vi "Message Handler (reentrant).vi"(7 "MsgQ Name":string, 8 "error in (no error)":errorcluster, 10 "Message to send":T1, 11 "Mode":T2) -> (0 "error out":errorcluster, 1 "Message Recieved?":bool, 2 "Message recieved":T1, 3 "Queue Names":string[](array[string]))   [LabVIEW 2013, in "Interloop MessageQ.lvlib"]
doc: "Keeps track of all message queues. Modes of operation : initialize, close, create queue, destroy queue, send message, Broadcase message (sends to queues excluding the passed in queue) read message. This vi should not block and controls access to messaging.\nReentrant must be wrapped for each message queue used in an application. Wrapper allows for create, send to read from, kill and broadcast."
uses:
  Interloop MessageQ.lvlib
  Message queue handler mode enums.ctl
  Message cluster.ctl
  Message Queue Ref.ctl
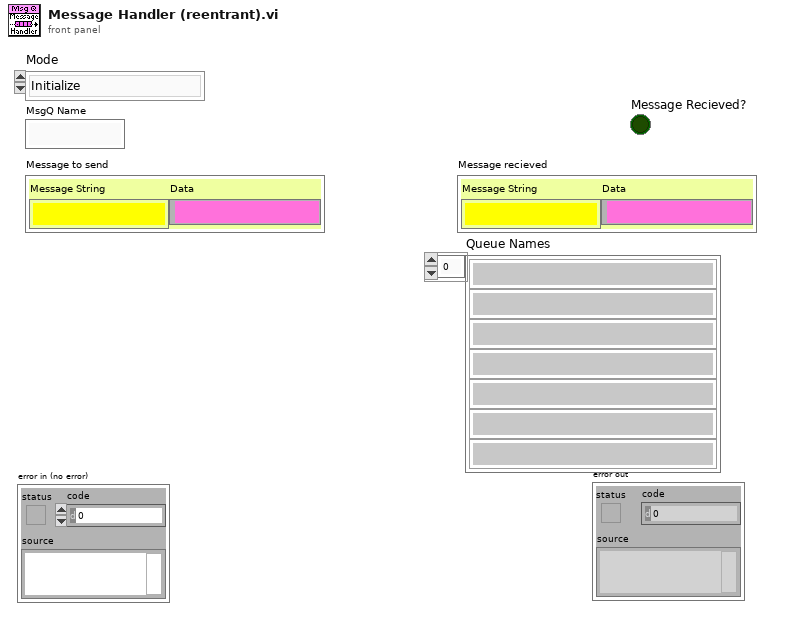
[diagram p1: front panel]
types:
  T1 = typedef "Interloop MessageQ.lvlib/Message cluster.ctl" = cluster{"Message String":string, "Data":variant}
  T2 = typedef "Interloop MessageQ.lvlib/Message queue handler mode enums.ctl" = enum16{"Initialize", "Create MsgQ", "Destroy MsgQ", "Send Message", "Broadcast Message", "Read Message", "Close"}
  T3 = typedef "Interloop MessageQ.lvlib/Message Queue Ref.ctl" = refnum<queue>
  T4 = typedef "Message cluster.ctl" = cluster{"Message String":string, "Data":variant}
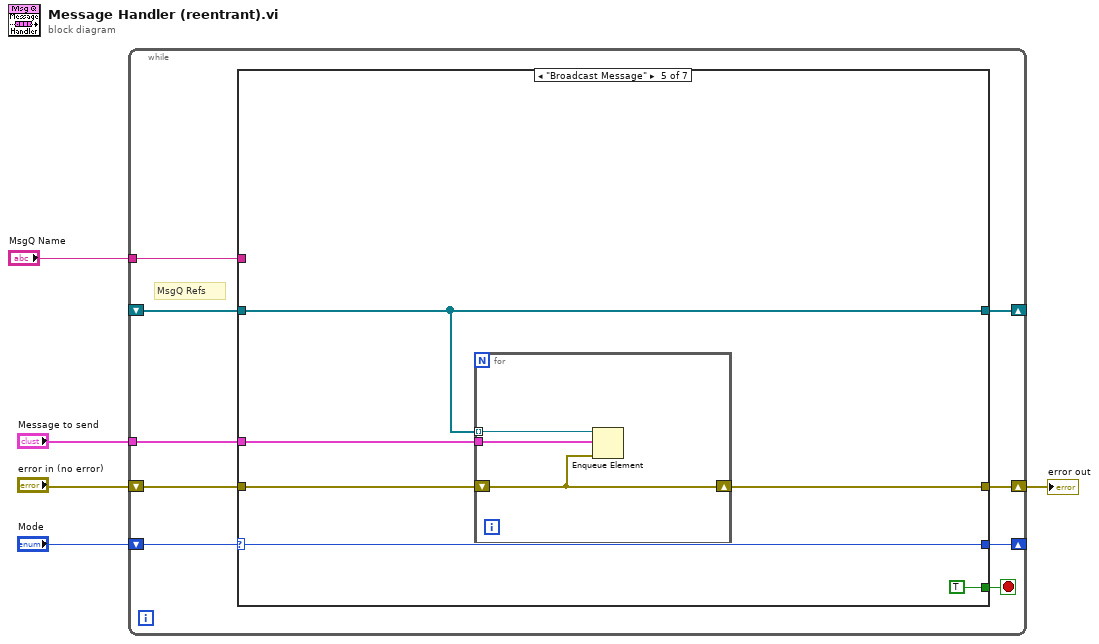
[diagram p0: block diagram]
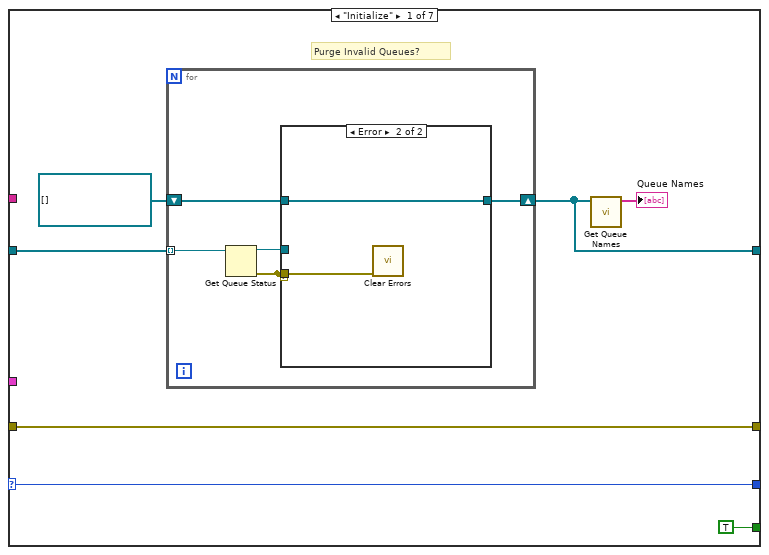
[diagram p2: hidden frame]
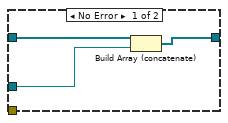
[diagram p3: hidden frame]
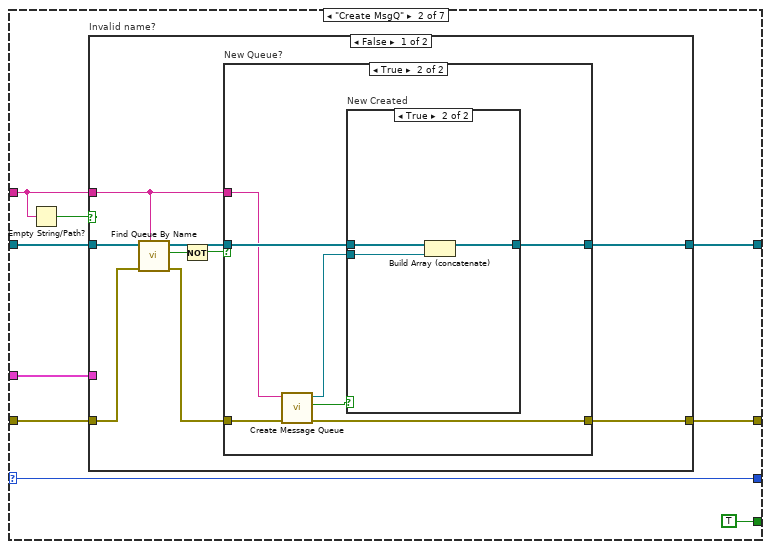
[diagram p4: hidden frame]
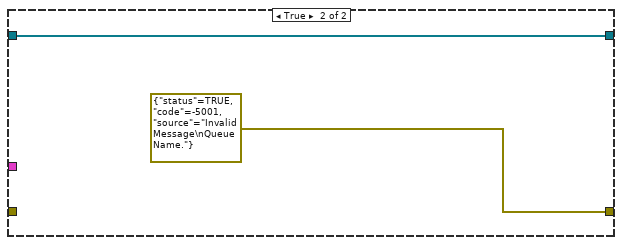
[diagram p7: hidden frame]
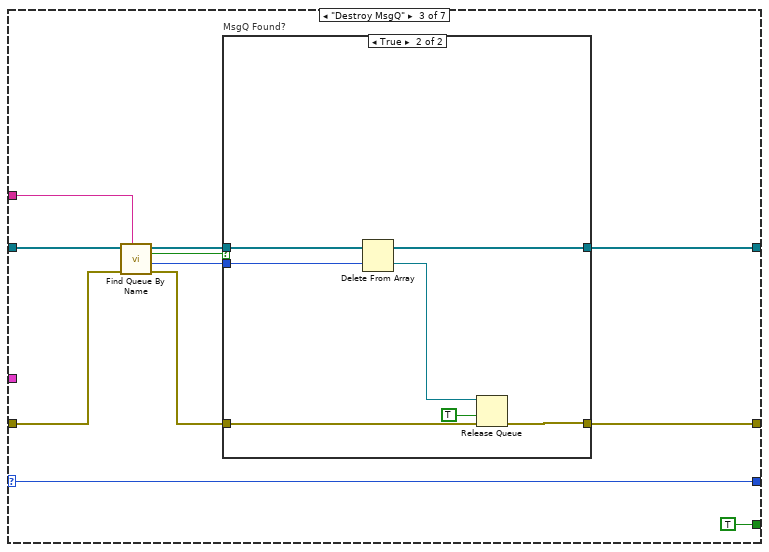
[diagram p8: hidden frame]
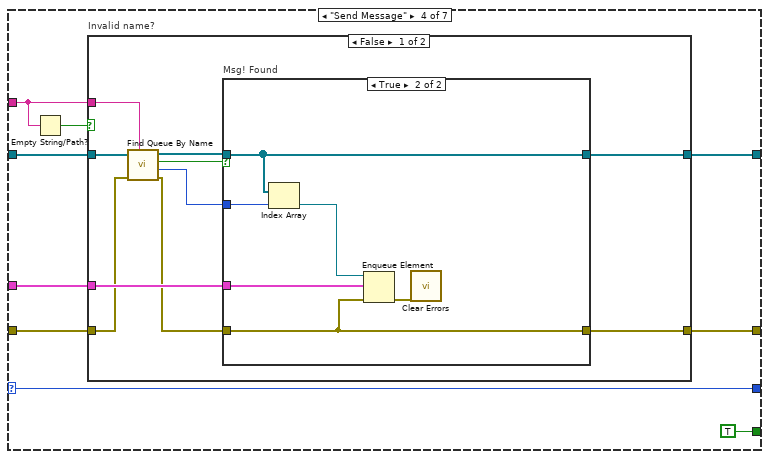
[diagram p10: hidden frame]
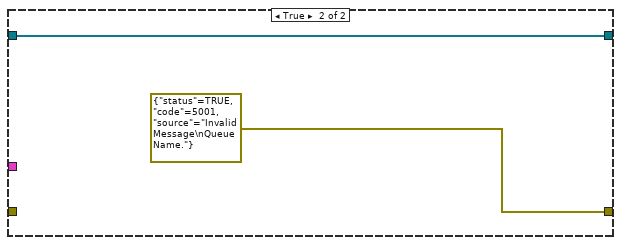
[diagram p12: hidden frame]
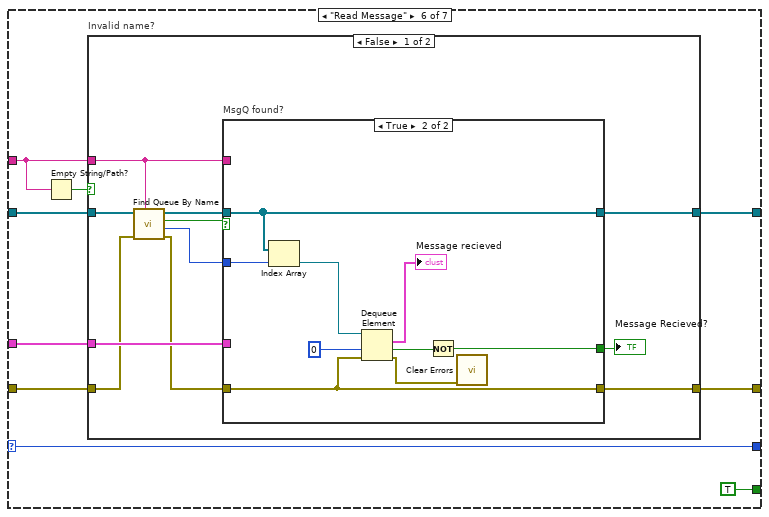
[diagram p13: hidden frame]
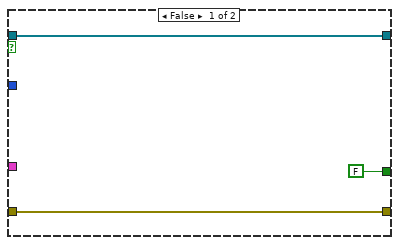
[diagram p14: hidden frame]
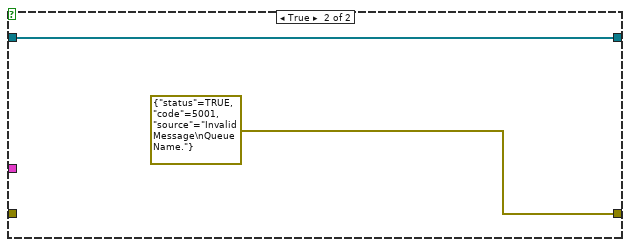
[diagram p15: hidden frame]
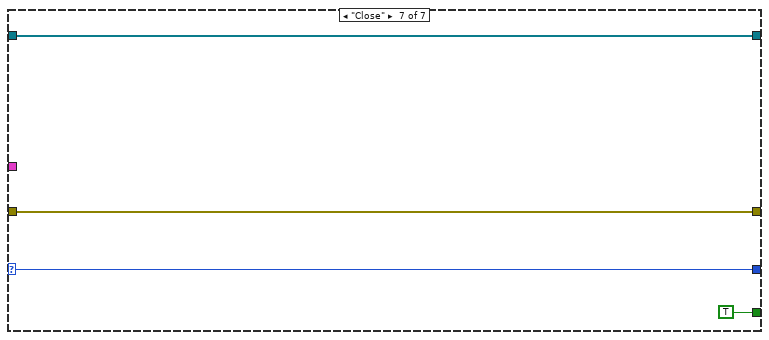
[diagram p16: hidden frame]
diagram:
  n1 = while {
    shift-right: [w13] -> _
    shift-left: _ -> [w12]
    shift-right: [w10] -> w5
    shift-left: "error in (no error)" -> [w11]
    tunnel: "MsgQ Name" -> [w9]
    shift-right: [w7] -> _
    shift-left: "Mode" -> [w14]
    tunnel: "Message to send" -> [w6]
    stop <- w8 stop-if-true
    # "MsgQ Refs"
    n2 = case shown="\"Broadcast Message\"" w14 {
      selector: w14 -> [w20 w37 w73 w90 w117 w128 w159]
      tunnel: [w16 w33 w72 w86 w114 w124 w157] -> w13
      tunnel: w12 -> [w18 w34 w71 w87 w114 w125 w157]
      tunnel: w11 -> [w19 w40 w70 w93 w119 w131 w160]
      tunnel: [w19 w39 w75 w92 w115 w130 w160] -> w10
      tunnel: w9 -> [_ w35 w65 w88 _ w126 _]
      tunnel: [TRUE TRUE TRUE TRUE TRUE TRUE TRUE] -> w8
      tunnel: [w20 w37 w73 w90 w117 w128 w159] -> w7
      tunnel: w6 -> [_ w32 _ w85 w116 w123 _]
      frame "Initialize" {
        # "Purge Invalid Queues?"
        n3 = for {
          tunnel: w18 -> [w26] mode=indexing
          shift-right: [w23] -> w16
          shift-left: T3[] [] ("Queue references out") -> [w24]
          n4 = Get Queue Status(queue=w26) -> (queue out=w25:T3, error out=w22:errorcluster)  [unwired: 1 in, 7 out]
          n5 = case shown="Error" w22 {
            tunnel: w25 -> [w28 _]
            tunnel: w24 -> [w29 w31]
            tunnel: [w27 w31] -> w23
            tunnel: w22 -> [_ w30]
            frame No Error {
              n6 = Build Array (concatenate)(w29, w28) -> (w27:T3[])
            }
            frame Error {
              n7 = call <vilib>:"Clear Errors.vi"("error in (no error)"=w30) -> ()  [unwired: 7 out]
            }
          }
        }
        n8 = call "Get Queue Names.vi"("Queue references"=w16) -> ("Queue Names"=→"Queue Names":string[])  [unwired: 10 out]
      }
      frame "Create MsgQ" {
        n9 = Empty String/Path?(string/path=w35) -> (empty?=w36:bool)
        n10 = case "Invalid name?" shown="False" w36 {
          tunnel: w40 -> [w45 _]
          tunnel: [w49 errorcluster {"status"=TRUE, "code"=-5001, "source"="Invalid Message\nQueue Name."} ("error out")] -> w39
          tunnel: w35 -> [w46 _]
          tunnel: w34 -> [w47 w64]
          tunnel: [w48 w64] -> w33
          tunnel: w32 -> [_ _]
          frame False {
            n11 = call "Find Queue By Name.vi"("MsgQ Name"=w46, "error in (no error)"=w45, "Queue references"=w47) -> ("error out"=w44:errorcluster, "Queue Found"=w41:bool, "Queue references out"=w42:T3[])  [unwired: 6 out]
            n12 = Not(x=w41) -> (.not. x?=w43:bool)
            n13 = case "New Queue?" shown="True" w43 {
              tunnel: w44 -> [w50 w58]
              tunnel: [w50 w57] -> w49
              tunnel: w46 -> [_ w52]
              tunnel: w42 -> [w51 w54]
              tunnel: [w51 w53] -> w48
              frame False {
              }
              frame True {
                n14 = call "Create Message Queue.vi"("error in (no error)"=w58, "Queue Name"=w52) -> ("error out"=w57:errorcluster, "created new?"=w56:bool, "queue ref out"=w55:T3)  [unwired: 2 in, 5 out]
                n15 = case "New Created" shown="True" w56 {
                  tunnel: w55 -> [_ w61]
                  tunnel: w54 -> [w59 w62]
                  tunnel: [w59 w60] -> w53
                  frame False {
                  }
                  frame True {
                    n16 = Build Array (concatenate)(w62, w61) -> (w60:T3[])
                  }
                }
              }
            }
          }
          frame True {
          }
        }
      }
      frame "Destroy MsgQ" {
        n17 = call "Find Queue By Name.vi"("MsgQ Name"=w65, "error in (no error)"=w70, "Queue references"=w71) -> ("error out"=w69:errorcluster, "Queue Index"=w68:i32, "Queue Found"=w67:bool, "Queue references out"=w66:T3[])  [unwired: 5 out]
        n18 = case "MsgQ Found?" shown="True" w67 {
          tunnel: w69 -> [w76 w83]
          tunnel: [w76 w80] -> w75
          tunnel: w66 -> [w77 w82]
          tunnel: [w77 w84] -> w72
          tunnel: w68 -> [_ w79]
          frame False {
          }
          frame True {
            n19 = Delete From Array(array=w82, index=w79) -> (deleted portion=w78:T3, array with subset deleted=w84:T3[])  [unwired: 1 in]
            n20 = Release Queue(queue=w78, force destroy? (F)=TRUE, error in (no error)=w83) -> (error out=w80:errorcluster)  [unwired: 2 out]
          }
        }
      }
      frame "Send Message" {
        n21 = Empty String/Path?(string/path=w88) -> (empty?=w89:bool)
        n22 = case "Invalid name?" shown="False" w89 {
          tunnel: w93 -> [w97 _]
          tunnel: [w103 errorcluster {"status"=TRUE, "code"=5001, "source"="Invalid Message\nQueue Name."} ("error out")] -> w92
          tunnel: w88 -> [w98 _]
          tunnel: w87 -> [w100 w113]
          tunnel: [w102 w113] -> w86
          tunnel: w85 -> [w101 _]
          frame False {
            n23 = call "Find Queue By Name.vi"("MsgQ Name"=w98, "error in (no error)"=w97, "Queue references"=w100) -> ("error out"=w96:errorcluster, "Queue Index"=w95:i32, "Queue Found"=w94:bool, "Queue references out"=w99:T3[])  [unwired: 5 out]
            n24 = case "Msg! Found" shown="True" w94 {
              tunnel: w96 -> [w104 w107]
              tunnel: [w104 w107] -> w103
              tunnel: w99 -> [w105 w111]
              tunnel: [w105 w111] -> w102
              tunnel: w95 -> [_ w110]
              tunnel: w101 -> [_ w108]
              frame False {
              }
              frame True {
                n25 = Index Array(array=w111, index=w110) -> (element=w109:T3)
                n26 = Enqueue Element(queue=w109, element=w108, error in (no error)=w107) -> (error out=w106:errorcluster)  [unwired: 3 out]
                n27 = call <vilib>:"Clear Errors.vi"("error in (no error)"=w106) -> ()  [unwired: 7 out]
              }
            }
          }
          frame True {
          }
        }
      }
      frame "Broadcast Message" {
        n28 = for {
          tunnel: w116 -> [w122]
          shift-right: [w120] -> w115
          shift-left: w119 -> [w120]
          tunnel: w114 -> [w121] mode=indexing
          n29 = Enqueue Element(queue=w121, element=w122, error in (no error)=w120) -> ()  [unwired: 4 out]
        }
      }
      frame "Read Message" {
        n30 = Empty String/Path?(string/path=w126) -> (empty?=w127:bool)
        n31 = case "Invalid name?" shown="False" w127 {
          tunnel: w131 -> [w134 _]
          tunnel: [w142 errorcluster {"status"=TRUE, "code"=5001, "source"="Invalid Message\nQueue Name."} ("error out")] -> w130
          tunnel: w126 -> [w133 _]
          tunnel: w125 -> [w138 w156]
          tunnel: [w141 w156] -> w124
          tunnel: w123 -> [w140 _]
          frame False {
            n32 = call "Find Queue By Name.vi"("MsgQ Name"=w133, "error in (no error)"=w134, "Queue references"=w138) -> ("error out"=w135:errorcluster, "Queue Index"=w137:i32, "Queue Found"=w132:bool, "Queue references out"=w136:T3[])  [unwired: 5 out]
            n33 = case "MsgQ found?" shown="True" w132 {
              tunnel: w135 -> [w144 w147]
              tunnel: [w144 w147] -> w142
              tunnel: w133 -> [_ _]
              tunnel: w136 -> [w145 w154]
              tunnel: [w145 w154] -> w141
              tunnel: w137 -> [_ w153]
              tunnel: w140 -> [_ _]
              tunnel: [FALSE w148] -> w139
              frame False {
              }
              frame True {
                n34 = Index Array(array=w154, index=w153) -> (element=w152:T3)
                n35 = Dequeue Element(queue=w152, timeout in ms (-1)=0, error in (no error)=w147) -> (element=→"Message recieved":T4, timed out?=w149:bool, error out=w146:errorcluster)  [unwired: 1 out]
                n36 = Not(x=w149) -> (.not. x?=w148:bool)
                n37 = call <vilib>:"Clear Errors.vi"("error in (no error)"=w146) -> ()  [unwired: 7 out]
              }
            }
            "Message Recieved?" <- w139
          }
          frame True {
          }
        }
      }
      frame "Close" {
      }
    }
  }
  "error out" <- w5
